vi "Convert Raw Data to DTCs.vi"(1 "data in":u8[](array[numeric]), 2 "DTC descriptor":T2={"DTC Byte Length"=2, "Status Byte Length"=1, "Add Data Byte Length"=0, "Byte Order"=enum."Motorola"}) -> (0 "DTCs":T1[](array[typedef]))   [LabVIEW 2019, in "GMLAN.lvlib"]
uses:
  GMLAN.lvlib
  <vilib>/Automotive Diagnostic Command Set/Diagnostic Protocols.llb/Diagnostic Trouble Code.ctl
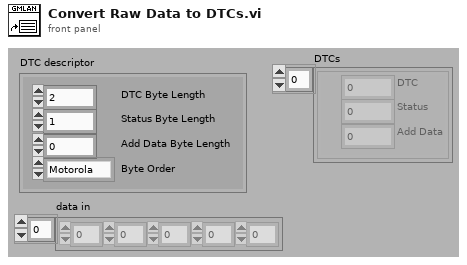
[diagram p1: front panel]
types:
  T1 = typedef "Diagnostic Trouble Code.ctl" = cluster{"DTC":u32, "Status":u32, "Add Data":u32}
  T2 = cluster{"DTC Byte Length":i32, "Status Byte Length":i32, "Add Data Byte Length":i32, "Byte Order":enum16{"Motorola", "Intel"}}
  T3 = cluster{"Start Byte":i32, "Byte Length":i32, "Byte Order":enum16{"Motorola", "Intel"}, "Data Type":enum16{"Unsigned", "Signed", "Float"}, "Scale Factor":dbl, "Scale Offset":dbl}
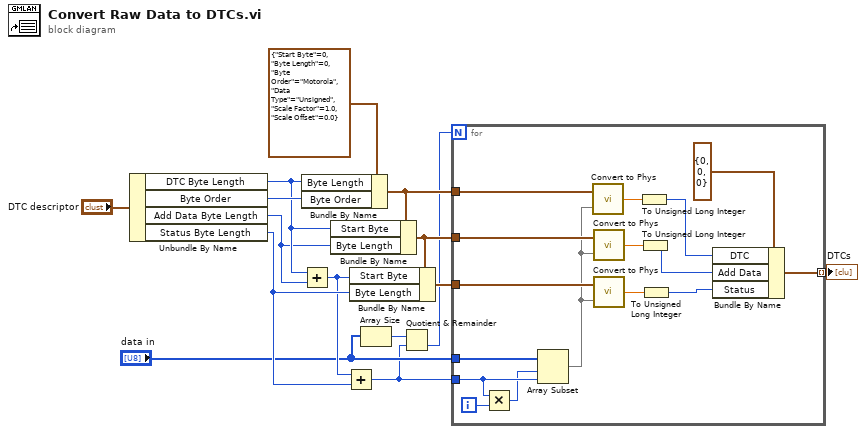
[diagram p0: block diagram]
diagram:
  n1 = Unbundle By Name("DTC descriptor") -> ("DTC Byte Length"=w7:i32, "Byte Order"=w8:enum16{"Motorola", "Intel"}, "Add Data Byte Length"=w6:i32, "Status Byte Length"=w12:i32)
  n2 = Bundle By Name(cluster=T3 {"Start Byte"=0, "Byte Length"=0, "Byte Order"=enum."Motorola", "Data Type"=enum."Unsigned", "Scale Factor"=1.0, "Scale Offset"=0.0} ("type descriptor"), "Byte Length"=w7, "Byte Order"=w8) -> (w9:T3)
  n3 = Add(x=w7, y=w6) -> (x+y=w5:i32)
  n4 = Bundle By Name(cluster=w9, "Start Byte"=w7, "Byte Length"=w6) -> (w14:T3)
  n5 = Add(x=w5, y=w12) -> (x+y=w2:i32)
  n6 = Bundle By Name(cluster=w14, "Start Byte"=w5, "Byte Length"=w12) -> (w13:T3)
  n7 = Array Size(array="data in") -> (size(s)=w3:i32)
  n8 = Quotient & Remainder(x=w3, y=w2) -> (floor(x/y)=w1:i32)  [unwired: 1 out]
  n9 = for {
    N: w1 -> [_]
    tunnel: w14 -> [w31]
    tunnel: w13 -> [w30]
    tunnel: "data in" -> [w27]
    tunnel: w2 -> [w25]
    tunnel: [w24] -> w11 mode=indexing
    tunnel: w9 -> [w22]
    i -> [w26]
    n10 = Multiply(x=w25, y=w26) -> (x*y=w19:i32)
    n11 = Array Subset(array=w27, index=w19, length=w25) -> (w21:u8[])
    n12 = call <vilib>:"Convert to Phys.vi"("data in"=w21, "type descriptor"=w22) -> ("value"=w20:dbl)
    n13 = call <vilib>:"Convert to Phys.vi"("data in"=w21, "type descriptor"=w31) -> ("value"=w29:dbl)
    n14 = call <vilib>:"Convert to Phys.vi"("data in"=w21, "type descriptor"=w30) -> ("value"=w28:dbl)
    n15 = To Unsigned Long Integer(number=w20) -> (unsigned 32bit integer=w18:u32)
    n16 = To Unsigned Long Integer(number=w29) -> (unsigned 32bit integer=w16:u32)
    n17 = To Unsigned Long Integer(number=w28) -> (unsigned 32bit integer=w17:u32)
    n18 = Bundle By Name(cluster=T1 {"DTC"=0, "Status"=0, "Add Data"=0} ("Diagnostic Trouble Code"), "DTC"=w18, "Add Data"=w16, "Status"=w17) -> (w24:T1)
  }
  "DTCs" <- w11
